vi "Rohde & Schwarz VNA Read Identification.vi"(8 "error in (no error)":errorcluster, 11 "VISA Resource Name":refnum<visa-resource-name>) -> (0 "error out":errorcluster, 1 "Serial Number":string, 2 "Model Number":string, 3 "dup VISA Resource Name":refnum<visa-resource-name>, 5 "Firmware":string)   [LabVIEW 2011]
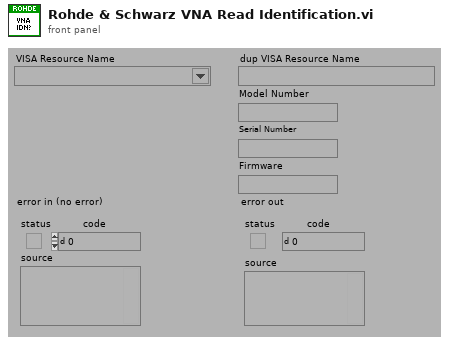
[diagram p1: front panel]
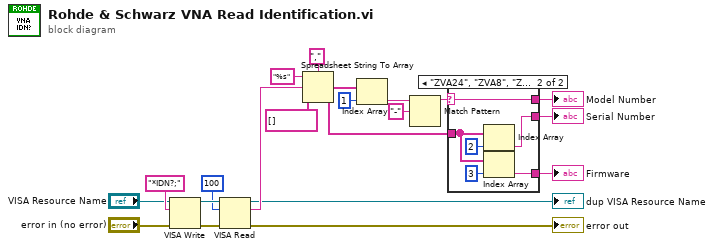
[diagram p0: block diagram]
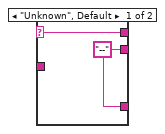
[diagram p2: hidden frame]
diagram:
  n1 = VISA Write(VISA resource name="VISA Resource Name", write buffer="*IDN?;", error in (no error)="error in (no error)") -> (VISA resource name out=w20:refnum<visa-resource-name>, error out=w18:errorcluster)  [unwired: 1 out]
  n2 = VISA Read(VISA resource name=w20, byte count=u32 100, error in (no error)=w18) -> (VISA resource name out=→"dup VISA Resource Name":refnum<visa-resource-name>, read buffer=w13:string, error out=→"error out":errorcluster)  [unwired: 1 out]
  n3 = Spreadsheet String To Array(delimiter (Tab)=",", format string="%s", spreadsheet string=w13, array type (2D Dbl)=string[] []) -> (array=w11:string[])
  n4 = Index Array(array=w11, index=1) -> (element=w2:string)
  n5 = Match Pattern(string=w2, regular expression="-") -> (before substring=w1:string)  [unwired: 4 out]
  n6 = case shown="\"ZVA24\", \"ZVA8\", \"ZVB20\", \"ZVB4\", \"ZVB8\", \"ZVT8\"" w1 {
    selector: w1 -> [w22 w28]
    tunnel: [w22 w28] -> w7
    tunnel: w11 -> [_ w23]
    tunnel: [w21 w26] -> w6
    tunnel: [w21 w24] -> w5
    frame "Unknown", Default {
      w21 = "--"
    }
    frame "ZVA24", "ZVA8", "ZVB20", "ZVB4", "ZVB8", "ZVT8" {
      n7 = Index Array(array=w23, index=2) -> (element=w26:string)
      n8 = Index Array(array=w23, index=3) -> (element=w24:string)
    }
  }
  "Model Number" <- w7
  "Serial Number" <- w6
  "Firmware" <- w5
